vi "DROPBEAR_Model_Updating_FFT.vi"(8 "error in (no error)":errorcluster, 11 "DROPBEAR_Model_Updating in":refnum<class "DROPBEAR_Model_Updating.lvclass">=refnum) -> (0 "error out":errorcluster, 3 "DROPBEAR_Model_Updating out":refnum<class "DROPBEAR_Model_Updating.lvclass">, 4 "looping":bool)   [LabVIEW 2021, in "DROPBEAR_Model_Updating.lvclass"]
uses:
  DROPBEAR_Model_Updating.lvclass
  MOCKBEAR/MOCKBEAR.lvclass
  FEA_Model/FEA_Model.lvclass
  Kalman_Filter/Kalman_Filter.lvclass
  Data_Array/Data_Array.lvclass
  Moving_Statistic/Moving_Statistic.lvclass
  Online_Statistic/Online_Statistic.lvclass
  Online_SNR/Online_SNR.lvclass
  Online_TRAC/Online_TRAC.lvclass
  DROPBEAR_Model_Updating.lvclass/DROPBEAR_Model_Updating.ctl
  Read FFT Bounding.vi
  <vilib>/Analysis/4window.llb/Hanning Window (DBL).vi
  <vilib>/Analysis/5stat.llb/RMS (DBL).vi
  <vilib>/Analysis/2dsp.llb/Real FFT.vi
  Write Time Cycle Start.vi
  Write Time Data Acquire.vi
  Write Time FFT.vi
  <vilib>/Analysis/4window.llb/AllCosWindow (DBL).vi
  <vilib>/Analysis/NI_AALPro.lvlib
panel:
  in  "Bound to 1st Frequency":bool=TRUE
  in  "Frequency Method":T1(ring)=enum."FFT"
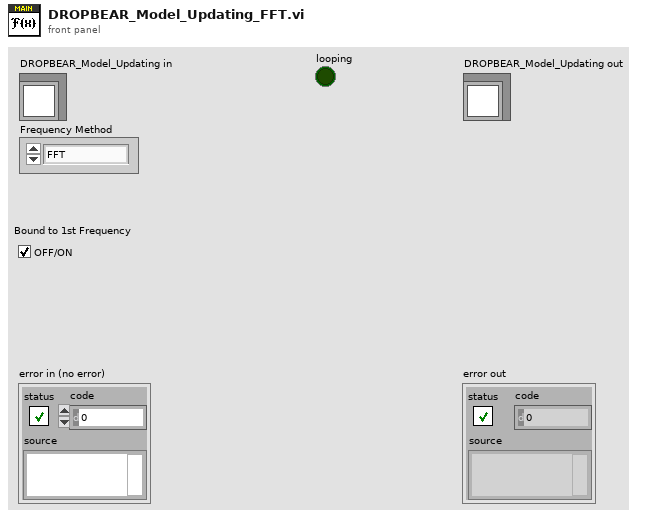
[diagram p1: front panel]
types:
  T1 = enum16{"Bandpass FFT", "Tone", "FFT", "Custom Filter"}
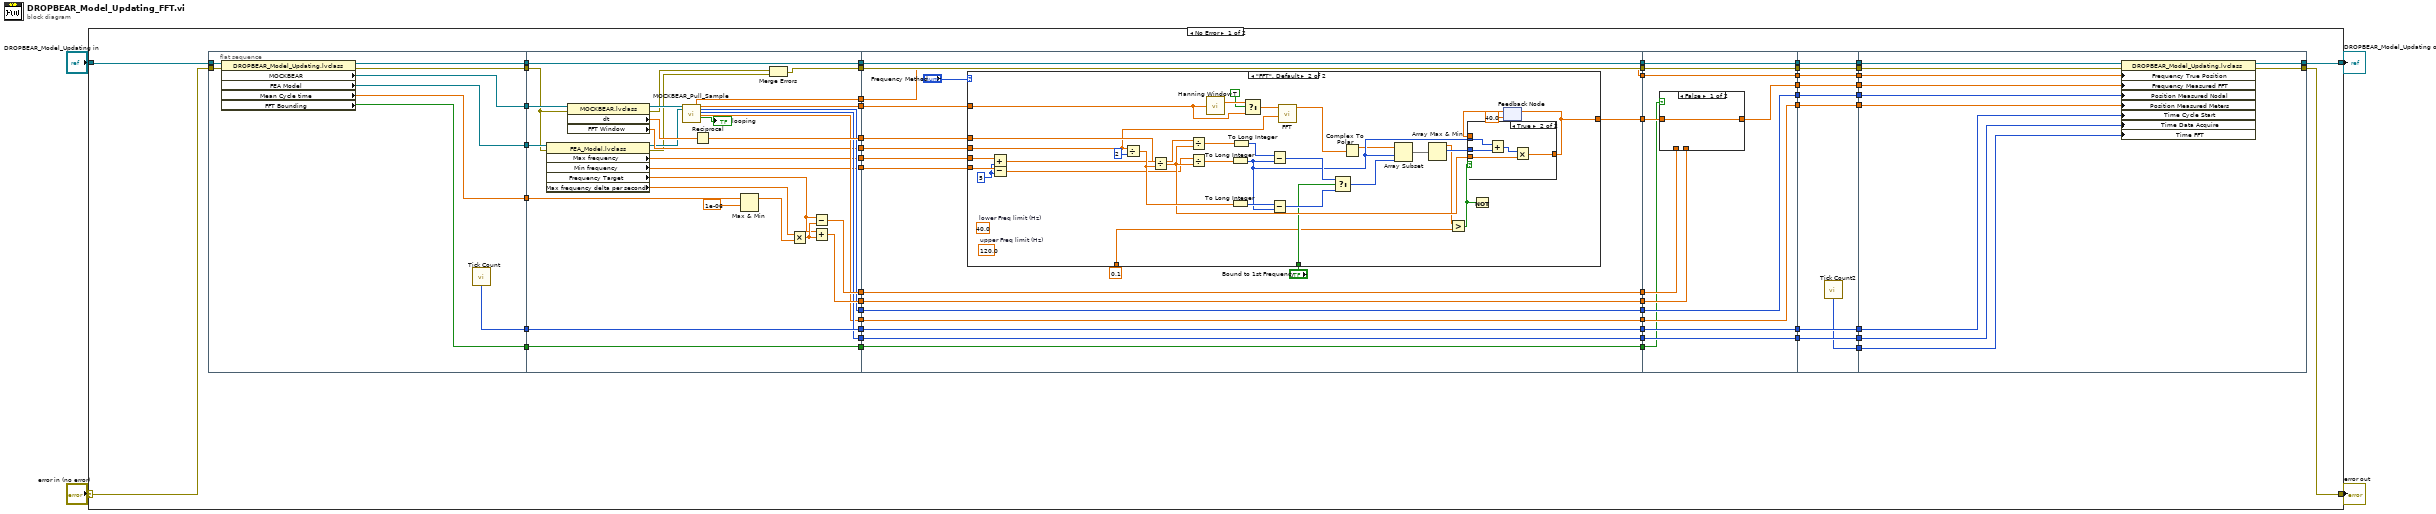
[diagram p0: block diagram]
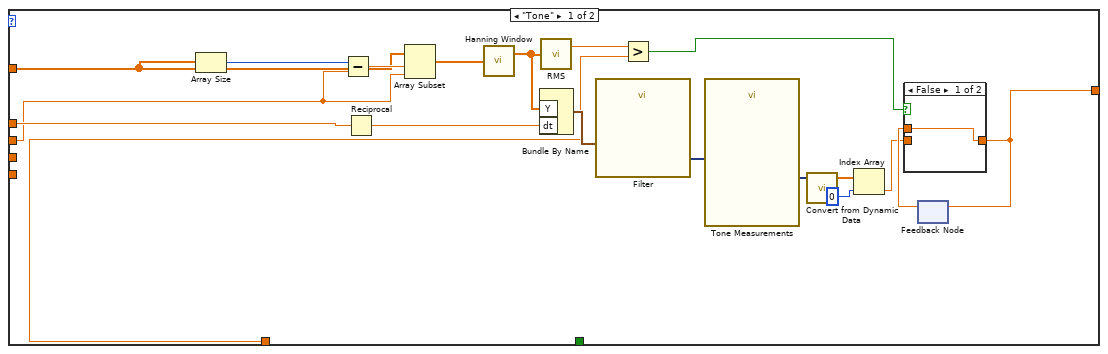
[diagram p2: hidden frame]
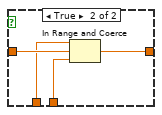
[diagram p5: hidden frame]
diagram:
  n1 = case shown="No Error" "error in (no error)" {
    selector: "error in (no error)" -> [w15 w215]
    tunnel: [w44 w214] -> w2
    tunnel: "DROPBEAR_Model_Updating in" -> [w33 w214]
    tunnel: [w9 w215] -> w1
    frame No Error {
      n2 = flat-sequence {
        tunnel: w33 -> [w66]
        tunnel: [w62] -> w58
        tunnel: [w64] -> w57
        tunnel: [w67] -> w40
        tunnel: [w65] -> w32
        tunnel: [w63] -> w23
        tunnel: [w61] -> w18
        tunnel: w15 -> [w60]
        tunnel: [w59] -> w14
        tunnel: w58 -> [w80]
        tunnel: w57 -> [w83]
        tunnel: [w94] -> w56
        tunnel: [w79] -> w55
        tunnel: [w78] -> w54
        tunnel: [w93] -> w53
        tunnel: [w81] -> w52
        tunnel: [w92] -> w51
        tunnel: [w91] -> w50
        tunnel: w40 -> [w90]
        tunnel: [w90] -> w39
        tunnel: [w89] -> w38
        tunnel: w32 -> [w88]
        tunnel: [w85] -> w31
        tunnel: [w84] -> w30
        tunnel: w23 -> [w74]
        tunnel: [w74] -> w22
        tunnel: w18 -> [w73]
        tunnel: [w73] -> w17
        tunnel: w14 -> [w72]
        tunnel: [w71] -> w10
        tunnel: [w68] -> w8
        tunnel: w56 -> [w113]
        tunnel: w55 -> [w112]
        tunnel: w54 -> [w111]
        tunnel: w53 -> [w114]
        tunnel: w52 -> [w109]
        tunnel: w51 -> [w116]
        tunnel: w50 -> [w115]
        tunnel: [w116] -> w49
        tunnel: [w115] -> w48
        tunnel: [w108] -> w47
        tunnel: [w105] -> w42
        tunnel: w39 -> [w105]
        tunnel: w38 -> [w104]
        tunnel: [w104] -> w35
        tunnel: w31 -> [w103]
        tunnel: w30 -> [w102]
        tunnel: [w103] -> w29
        tunnel: [w102] -> w28
        tunnel: w22 -> [w101]
        tunnel: [w101] -> w21
        tunnel: w17 -> [w100]
        tunnel: [w100] -> w16
        tunnel: [w99] -> w13
        tunnel: w10 -> [w99]
        tunnel: w8 -> [w98]
        tunnel: [w98] -> w6
        tunnel: w49 -> [w186]
        tunnel: w48 -> [w187]
        tunnel: w47 -> [w188]
        tunnel: [w185] -> w46
        tunnel: w42 -> [w184]
        tunnel: [w184] -> w41
        tunnel: [w183] -> w37
        tunnel: w35 -> [w183]
        tunnel: w29 -> [w182]
        tunnel: w28 -> [w181]
        tunnel: [w182] -> w26
        tunnel: [w181] -> w25
        tunnel: w21 -> [w180]
        tunnel: [w180] -> w20
        tunnel: w16 -> [w179]
        tunnel: w13 -> [w178]
        tunnel: [w178] -> w12
        tunnel: [w177] -> w7
        tunnel: w6 -> [w177]
        tunnel: w46 -> [w202]
        tunnel: [w202] -> w45
        tunnel: [w201] -> w43
        tunnel: w41 -> [w201]
        tunnel: w37 -> [w200]
        tunnel: [w200] -> w36
        tunnel: [w199] -> w34
        tunnel: [w198] -> w27
        tunnel: w26 -> [w198]
        tunnel: w25 -> [w197]
        tunnel: [w197] -> w24
        tunnel: w20 -> [w196]
        tunnel: [w196] -> w19
        tunnel: w12 -> [w195]
        tunnel: [w195] -> w11
        tunnel: w7 -> [w194]
        tunnel: [w194] -> w5
        tunnel: w45 -> [w204]
        tunnel: [w211] -> w44
        tunnel: w43 -> [w209]
        tunnel: w36 -> [w208]
        tunnel: w34 -> [w207]
        tunnel: w27 -> [w213]
        tunnel: w24 -> [w212]
        tunnel: w19 -> [w210]
        tunnel: w11 -> [w206]
        tunnel: [w205] -> w9
        tunnel: w5 -> [w203]
        frame #0 {
          n3 = property class="DROPBEAR_Model_Updating.lvclass"(reference=w66, error in=w60) -> (reference out=w63:refnum<class "DROPBEAR_Model_Updating.lvclass">, error out=w59:errorcluster, "MOCKBEAR"=w65:refnum<class "MOCKBEAR.lvclass">, "FEA Model"=w62:refnum<class "FEA_Model.lvclass">, "Mean Cycle time"=w64:dbl, "FFT Bounding"=w61:bool)
          n4 = call "Tick Count"() -> ("Tick Count(uSec)"=w67:u32)
        }
        frame #1 {
          n5 = property class="FEA_Model.lvclass"(reference=w80, error in=w72) -> (reference out=w75:refnum<class "FEA_Model.lvclass">, error out=w70:errorcluster, "Max frequency"=w79:dbl, "Min frequency"=w78:dbl, "Frequency Target"=w77:dbl, "Max frequency delta per second"=w76:dbl)
          n6 = property class="MOCKBEAR.lvclass"(reference=w88, error in=w72) -> (reference out=w86:refnum<class "MOCKBEAR.lvclass">, error out=w69:errorcluster, "dt"=w87:dbl, "FFT Window"=w81:dbl)
          n7 = call "MOCKBEAR_Pull_Sample.vi"("MOCKBEAR in"=w86, "FEA Model"=w75) -> ("Frequency True"=w68:dbl, "Accelerometer sample"=w93:dbl[], "Last pin pos node"=w85:i32, "Sample Time"=w89:u32, "Last pin pos meter"=w84:dbl, "looping"=→"looping":bool)  [unwired: 11 in, 1 out]
          n8 = Reciprocal(x=w87) -> (1/x=w94:dbl)
          n9 = Max & Min(x=w83, y=1e-06) -> (max(x,y)=w97:dbl)  [unwired: 1 out]
          n10 = Merge Errors(w69, w70) -> (w71:errorcluster)
          n11 = Multiply(x=w76, y=w97) -> (x*y=w96:dbl)
          n12 = Subtract(x=w77, y=w96) -> (x-y=w92:dbl)
          n13 = Add(x=w77, y=w96) -> (x+y=w91:dbl)
        }
        frame #2 {
          n14 = case shown="\"FFT\", Default" "Frequency Method" {
            tunnel: [w123 w146] -> w108
            tunnel: w114 -> [w127 w140]
            tunnel: "Bound to 1st Frequency" -> [_ w158]
            tunnel: w113 -> [w119 w150]
            tunnel: w112 -> [_ w147]
            tunnel: w111 -> [_ w143]
            tunnel: 0.1 -> [w117 w148]
            tunnel: w109 -> [w118 w149]
            frame "Tone" {
              n15 = Array Size(array=w127) -> (size(s)=w135:i32)
              n16 = Subtract(x=w135, y=w118) -> (x-y=w134:dbl)
              n17 = Reciprocal(x=w119) -> (1/x=w120:dbl)
              n18 = Array Subset(array=w127, index=w134, length=w118) -> (w128:dbl[])
              n19 = call-poly <vilib>:"Hanning Window.vi"("X"=w128) -> ("Windowed X"=w125:dbl[])  [unwired: 1 out]
              n20 = Bundle By Name("Y"=w125, "dt"=w120) -> (w129:waveform(dbl))  [unwired: 1 in]
              n21 = call-poly <vilib>:"RMS.vi"("X"=w125) -> ("rms value"=w121:dbl)  [unwired: 1 out]
              n22 = call "Filter"("Signal"=w129) -> ("Filtered Signal"=w130:dynamicdata)  [unwired: 9 in, 1 out]
              n23 = Greater?(x=w121, y=w117) -> (0:w122:bool)
              n24 = call "Tone Measurements"("Signals"=w130) -> ("Frequency"=w131:dynamicdata)  [unwired: 9 in, 1 out]
              n25 = call "Convert from Dynamic Data"("Dynamic Data Type"=w131) -> ("Array"=w132:dbl[])  [unwired: 3 in]
              n26 = Index Array(array=w132, index=0) -> (element=w124:dbl)
              n27 = feedback #1() -> (w126:dbl)  [unwired: 1 in]
              n28 = case shown="False" w122 {
                tunnel: [w136 w137] -> w123
                tunnel: w126 -> [w136 _]
                tunnel: w124 -> [_ w137]
                frame False {
                }
                frame True {
                }
              }
              n29 = feedback-in #1(w123) -> ()
            }
            frame "FFT", Default {
              w138 = 5 ("y")
              (unwired) 120.0  # upper Freq limit (Hz)
              (unwired) 40.0  # lower Freq limit (Hz)
              n30 = Add(x=w147, y=w138) -> (x+y=w152:dbl)
              n31 = Subtract(x=w143, y=w138) -> (x-y=w153:dbl)
              n32 = Divide(x=w149, y=2) -> (x/y=w166:dbl)
              n33 = Divide(x=w150, y=w166) -> (x/y=w164:dbl)
              n34 = Divide(x=w152, y=w164) -> (x/y=w163:dbl)
              n35 = Divide(x=w153, y=w164) -> (x/y=w169:dbl)
              n36 = call-poly <vilib>:"Hanning Window.vi"("X"=w140) -> ("Windowed X"=w142:dbl[])  [unwired: 1 out]
              n37 = To Long Integer(number=w169) -> (32bit integer=w154:i32)
              n38 = To Long Integer(number=w166) -> (32bit integer=w167:i32)
              n39 = To Long Integer(number=w163) -> (32bit integer=w162:i32)
              n40 = Select(t=w142, s=TRUE, f=w140) -> (s? t:f=w139:dbl[])
              n41 = Subtract(x=w162, y=w154) -> (x-y=w160:i32)
              n42 = Subtract(x=w167, y=w154) -> (x-y=w159:i32)
              n43 = call-poly <vilib>:"FFT.vi"("FFT size"=w149, "X"=w139) -> ("FFT {X}"=w157:cdb[])  [unwired: 8 in, 1 out]
              n44 = Select(t=w160, s=w158, f=w159) -> (s? t:f=w161:i32)
              n45 = Complex To Polar(r * e^(i*theta)=w157) -> (r=w145:dbl[])  [unwired: 1 out]
              n46 = Array Subset(array=w145, index=w154, length=w161) -> (w144:dbl[])
              n47 = Array Max & Min(array=w144) -> (max value=w151:dbl, max index (indices)=w168:i32)  [unwired: 2 out]
              n48 = Greater?(x=w151, y=w148) -> (0:w165:bool)
              n49 = Not(x=w165) -> ()  [unwired: 1 out]
              n50 = feedback #2(40.0) -> (w156:dbl)
              n51 = case shown="True" w165 {
                tunnel: w168 -> [_ w173]
                tunnel: w154 -> [_ w174]
                tunnel: w164 -> [_ w175]
                tunnel: [w171 w172] -> w146
                tunnel: w156 -> [w171 _]
                frame False {
                }
                frame True {
                  n52 = Add(x=w174, y=w173) -> (x+y=w176:i32)
                  n53 = Multiply(x=w176, y=w175) -> (x*y=w172:dbl)
                }
              }
              n54 = feedback-in #2(w146) -> ()
            }
          }
        }
        frame #3 {
          n55 = case shown="False" w179 {
            tunnel: w188 -> [w189 w193]
            tunnel: [w189 w192] -> w185
            tunnel: w187 -> [_ w190]
            tunnel: w186 -> [_ w191]
            frame False {
            }
            frame True {
              n56 = In Range and Coerce(upper limit=w191, x=w193, lower limit=w190) -> (coerced(x)=w192:dbl)  [unwired: 1 out]
            }
          }
        }
        frame #4 {
          n57 = call "Tick Count2"() -> ("Tick Count(uSec)"=w199:u32)
        }
        frame #5 {
          n58 = property class="DROPBEAR_Model_Updating.lvclass"(reference=w210, error in=w206, "Frequency True Position"=w203, "Frequency Measured FFT"=w204, "Position Measured Nodal"=w213, "Position Measured Meters"=w212, "Time Cycle Start"=w209, "Time Data Acquire"=w208, "Time FFT"=w207) -> (reference out=w211:refnum<class "DROPBEAR_Model_Updating.lvclass">, error out=w205:errorcluster)
        }
      }
    }
    frame Error {
    }
  }
  "error out" <- w1
  "DROPBEAR_Model_Updating out" <- w2
